vi "fft_demod_update.vi"(6 "Reset":bool, 10 "Config":T1={"I/O"={"Format"={"Rate"=4, "Bits"=32, "Channels"=2}, "card #"=1, "# buffers"=96000}, "High rate STFT"={"Win param"=101.5, "Window type"=61, "Win order"=2, "DFT size"=64, "Channels"=[7], "Oversample"=64}, "Low rate STFT"={"Win param"=120.0, "Window type"=61, "Win order"=8, "DFT size"=64, "Channels"=[7], "Oversample"=64}, "Filtering"={"Hum"={"Frequency"=0.0, "Tc"=0.0, "Limit"=101.5, "FFT filter"=FALSE, "Detrend mode"=enum."Robust linear", "Enable"=FALSE}, "Kalman"={"Process noise"=101.5, "Measure noise"=101.5, "Unlock m noise"=101.5, "Mode"=enum."FFT"}, "Distortion"={"LF cut"=101.5, "Tc"=3.0, "Limit"=101.5, "FFT filter"=FALSE, "Detrend mode"=enum."Robust linear", "Enable"=FALSE}, "Lowpass"={"Frequency"=0.0, "Order"=0, "Enable"=FALSE}, "Impulse"={"Win order"=102, "Locked limit"=101.5, "Locked count"=102, "Threshold Tc"=101.5, "Thresh sigmas"=101.5, "Thresh min"=101.5, "After"=0, "Detrend"=FALSE, "Enable"=FALSE}}} {"Filtering"."Impulse"."Thresh min" format="%#_3p"; "Filtering"."Impulse"."Threshold Tc" format="%#_3p"; "Filtering"."Impulse"."Locked limit" format="%#_3p"; "Filtering"."Impulse"."Thresh sigmas" format="%#_3p"; "Filtering"."Lowpass"."Frequency" format="%#_4p"; "Filtering"."Distortion"."Limit" format="%#_3p"; "Filtering"."Distortion"."LF cut" format="%#_3p"; "Filtering"."Kalman"."Unlock m noise" format="%#_3p"; "Filtering"."Kalman"."Measure noise" format="%#_3p"; "Filtering"."Kalman"."Process noise" format="%#_3p"; "Filtering"."Hum"."Limit" format="%#_3p"; "Filtering"."Hum"."Frequency" format="%#_4p"; "Low rate STFT"."Oversample" min=1 step=1; "Low rate STFT"."Channels" min=0 step=1; "Low rate STFT"."DFT size" min=1 step=1; "Low rate STFT"."Window type" items=["Rectangle"=0, "Hanning"=1, "Hamming"=2, "Blackman-Harris"=3, "Exact Blackman"=4, "Blackman"=5, "Flat Top"=6, "4 Term B-Harris "=7, "7 Term B-Harris"=8, "Low Sidelobe"=9, "Blackman Nuttall"=11, "Triangle"=30, "Bartlett-Hanning"=31, "Bohman"=32, "Parzen"=33, "Welch"=34, "Kaiser"=60, "Dolph-Chebyshev"=61, "Gaussian"=62]; "High rate STFT"."Oversample" min=1 step=1; "High rate STFT"."Channels" min=0 step=1; "High rate STFT"."DFT size" min=1 step=1; "High rate STFT"."Window type" items=["Rectangle"=0, "Hanning"=1, "Hamming"=2, "Blackman-Harris"=3, "Exact Blackman"=4, "Blackman"=5, "Flat Top"=6, "4 Term B-Harris "=7, "7 Term B-Harris"=8, "Low Sidelobe"=9, "Blackman Nuttall"=11, "Triangle"=30, "Bartlett-Hanning"=31, "Bohman"=32, "Parzen"=33, "Welch"=34, "Kaiser"=60, "Dolph-Chebyshev"=61, "Gaussian"=62]}, 11 "Signal":dbl[](array[numeric])) -> (0 "Measure noise covariance":dbl[](array[numeric]), 2 "Measurement amplitudes":cdb[](array[numeric]) format="%_3p")   [LabVIEW 2014]
uses:
  ilemt_config.ctl
  io_config.ctl
  stft_params.ctl
  <vilib>/Analysis/4window.llb/windowTd.ctl
  filter_params.ctl
  detrend_mode.ctl
  <vilib>/Analysis/NI_AALPro.lvlib
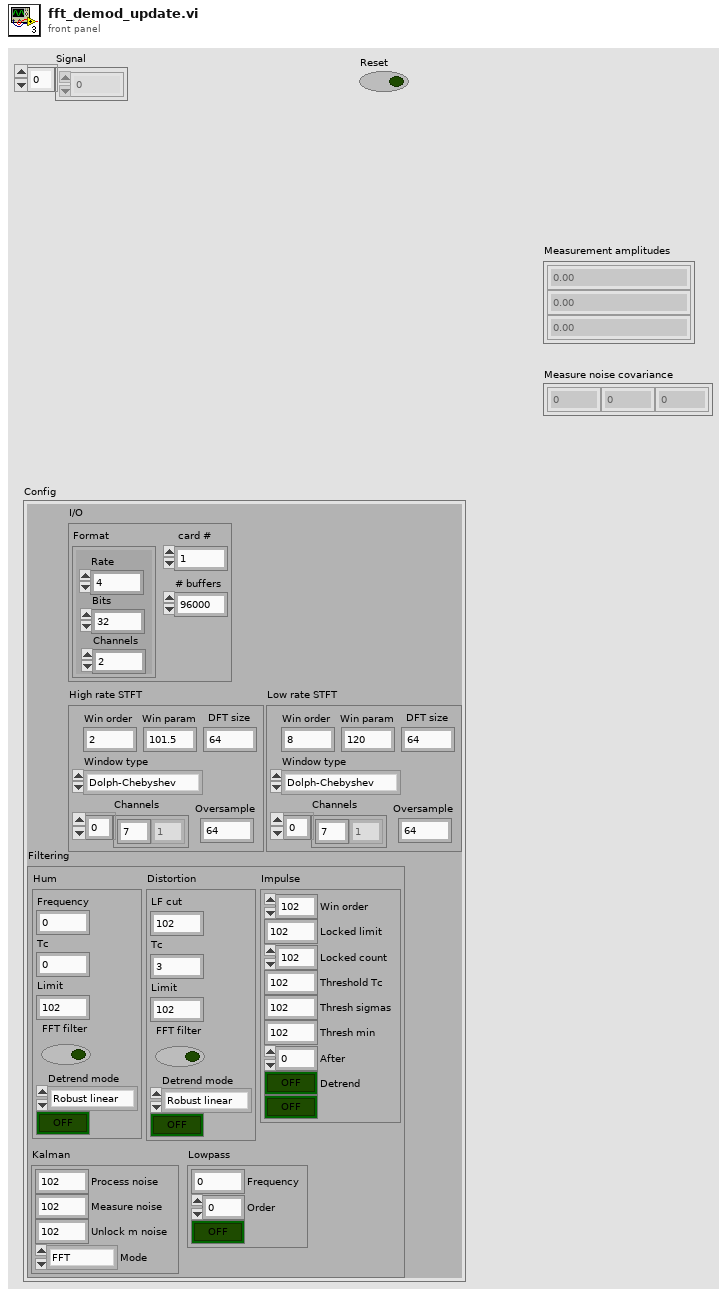
[diagram p1: front panel]
types:
  T1 = typedef "ilemt_config.ctl" = cluster{"I/O":T2, "High rate STFT":T3, "Low rate STFT":T3, "Filtering":T5}
  T2 = typedef "io_config.ctl" = cluster{"Format":cluster{"Rate":i32, "Bits":i32, "Channels":u32}, "card #":u32, "# buffers":i32}
  T3 = typedef "stft_params.ctl" = cluster{"Win param":dbl, "Window type":T4, "Win order":i32, "DFT size":i32, "Channels":i32[], "Oversample":i32}
  T4 = typedef "NI_AALPro.lvlib/windowTd.ctl" = u32
  T5 = typedef "filter_params.ctl" = cluster{"Hum":cluster{"Frequency":dbl, "Tc":dbl, "Limit":dbl, "FFT filter":bool, "Detrend mode":T6, "Enable":bool}, "Kalman":cluster{"Process noise":dbl, "Measure noise":dbl, "Unlock m noise":dbl, "Mode":enum16{"FFT", "KF demod"}}, "Distortion":cluster{"LF cut":dbl, "Tc":dbl, "Limit":dbl, "FFT filter":bool, "Detrend mode":T6, "Enable":bool}, "Lowpass":cluster{"Frequency":dbl, "Order":i32, "Enable":bool}, "Impulse":cluster{"Win order":i32, "Locked limit":dbl, "Locked count":i32, "Threshold Tc":dbl, "Thresh sigmas":dbl, "Thresh min":dbl, "After":i32, "Detrend":bool, "Enable":bool}}
  T6 = typedef "detrend_mode.ctl" = enum16{"Zero mean", "Linear", "Robust linear"}
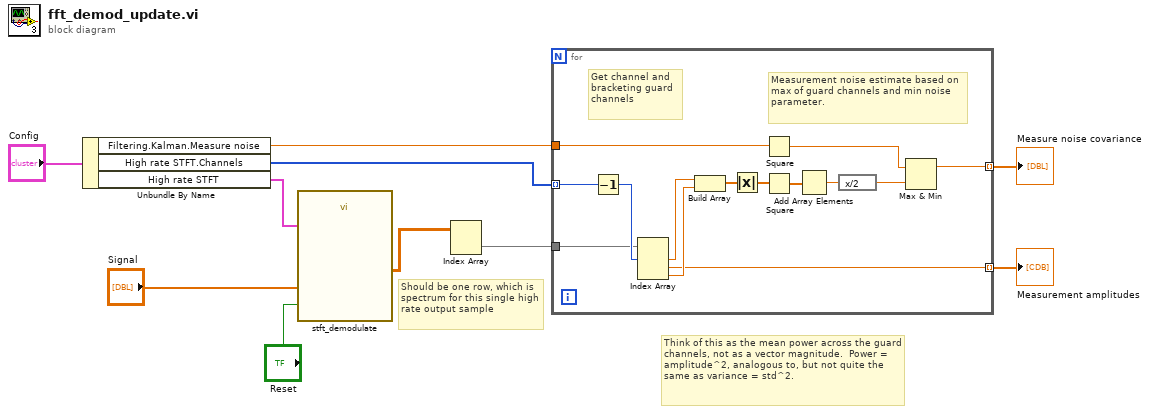
[diagram p0: block diagram]
diagram:
  # "Think of this as the mean power across the guard channels, not as a vector magnitude.  Power = amplitude^2, analogous to, but not quite the same as variance = std^2."
  # "Should be one row, which is spectrum for this single high rate output sample"
  n1 = Unbundle By Name("Config") -> ("Filtering.Kalman.Measure noise"=w7:dbl, "High rate STFT.Channels"=w5:i32[], "High rate STFT"=w8:T3)
  n2 = call "stft_demodulate.vi"("STFT params"=w8, "Reset"="Reset", "X"="Signal") -> ("STFT"=w4:cdb[][])  [unwired: 6 in, 2 out]
  n3 = Index Array(array=w4) -> (element=w3:cdb[])  [unwired: 2 in]
  n4 = for {
    tunnel: [w15] -> w1 mode=indexing
    tunnel: w3 -> [w12]
    tunnel: w5 -> [w13] mode=indexing
    tunnel: w7 -> [w18]
    tunnel: [w11] -> w2 mode=indexing
    # "Measurement noise estimate based on max of guard channels and min noise parameter."
    # "Get channel and bracketing guard channels"
    n5 = Decrement(x=w13) -> (x-1=w24:i32)
    n6 = Index Array(array=w12, index #1=w24) -> (element #1=w23:cdb, element #2=w15:cdb, element #3=w22:cdb)  [unwired: 2 in]
    n7 = Build Array(w23, w22) -> (w17:cdb[])
    n8 = Absolute Value(x=w17) -> (abs(x)=w16:dbl[])
    n9 = Square(x=w18) -> (x^2=w14:dbl)
    n10 = Square(x=w16) -> (x^2=w20:dbl[])
    n11 = Add Array Elements(numeric array=w20) -> (sum=w21:dbl)
    n12 = expression code="x/2"(w21) -> (w19:dbl)
    n13 = Max & Min(x=w14, y=w19) -> (max(x,y)=w11:dbl)  [unwired: 1 out]
  }
  "Measurement amplitudes" <- w1
  "Measure noise covariance" <- w2
